vi "UpdateViMult.vi"(8 "error in (no error)":errorcluster, 10 "dirOfCtrl":path, 11 "arrayOfVi":path[](array[path])) -> (0 "error out":errorcluster, 3 "arrayOfViRenamed":path[](array[path]))   [LabVIEW 2018]
doc: "Update the controls and names in multiple vi. The updated vi will be saved as a new file."
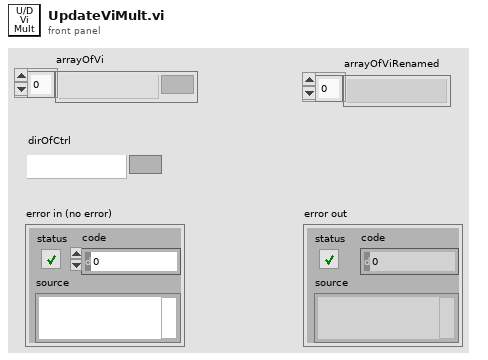
[diagram p1: front panel]
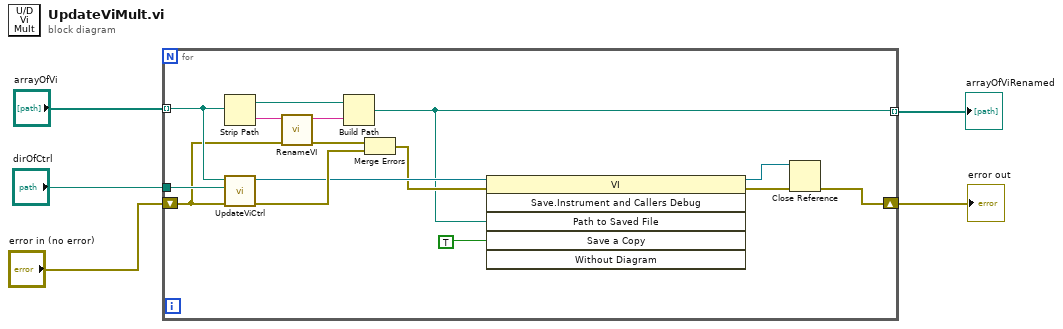
[diagram p0: block diagram]
diagram:
  n1 = for {
    tunnel: "arrayOfVi" -> [w19] mode=indexing
    tunnel: "dirOfCtrl" -> [w20]
    shift-right: [w7] -> w4
    shift-left: "error in (no error)" -> [w15]
    tunnel: [w9] -> w1 mode=indexing
    n2 = Strip Path(path=w19) -> (stripped path=w18:path, name=w17:string)
    n3 = call "UpdateViCtrl.vi"("error in (no error)"=w15, "Controls"=w20, "VIToUpdate"=w19) -> ("error out"=w13:errorcluster, "reference out"=w12:refnum<vi>)  [unwired: 7 in]
    n4 = call "RenameVI.vi"("error in (no error)"=w15, "InitialName"=w17) -> ("error out"=w14:errorcluster, "NewName"=w16:string)  [unwired: 8 in]
    n5 = Build Path(base path=w18, name or relative path=w16) -> (appended path=w9:path)
    n6 = Merge Errors(w14, w13) -> (w11:errorcluster)
    n7 = invoke class="VI" method="Save.Instrument and Callers Debug"(reference=w12, error in=w11, "Path to Saved File"=w9, "Save a Copy"=TRUE) -> (reference out=w6:refnum<vi>, error out=w8:errorcluster)  [unwired: 2 in, 4 out]
    n8 = Close Reference(reference=w6, error in (no error)=w8) -> (error out=w7:errorcluster)
  }
  "error out" <- w4
  "arrayOfViRenamed" <- w1
